vi "server start.vi"(8 "error in":errorcluster, 11 "run minimized (T)":bool=TRUE) -> (0 "error out":errorcluster)   [LabVIEW 2024]
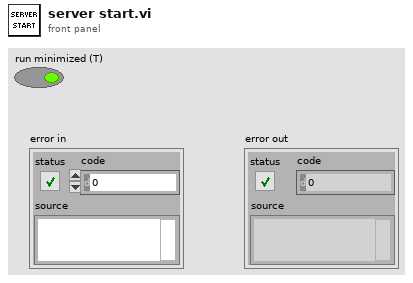
[diagram p1: front panel]
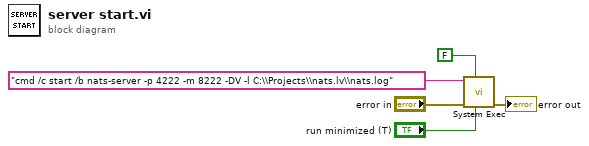
[diagram p0: block diagram]
diagram:
  n1 = call <vilib>:"System Exec.vi"("run minimized? (F)"="run minimized (T)", "wait until completion? (T)"=FALSE, "error in (no error)"="error in", "command line"="cmd /c start /b nats-server -p 4222 -m 8222 -DV -l C:\\Projects\\nats.lv\\nats.log") -> ("error out"=→"error out":errorcluster)  [unwired: 4 in, 3 out]
